vi "Create.vi"(8 "error in (no error)":errorcluster, 11 "ICPCON M7024 in":refnum<class "ICPCON M-7024.lvclass">) -> (0 "error out":errorcluster, 3 "ICPCON M7024 out":refnum<class "ICPCON M-7024.lvclass">)   [LabVIEW 2021, in "ICPCON M-7024.lvclass"]
uses:
  ICPCON M-7024.lvclass
  D:/my_projects/projects/Algorithms/Labview/21/Master CR/Master CR.lvclass
  Data Model/ICPCON ET7000 Data Model/M-7024/M-7024 Data Model.lvclass
  D:/my_projects/projects/Algorithms/Labview/21/Modbus_v121c/Data Model/Device Data Model.lvclass
  Master CR.lvclass/Master CR.ctl
  Serial/Modbus Serial/Modbus Serial.lvclass
  ICPCON M-7024.lvclass/ICPCON M-7024.ctl
  Master CR.lvclass
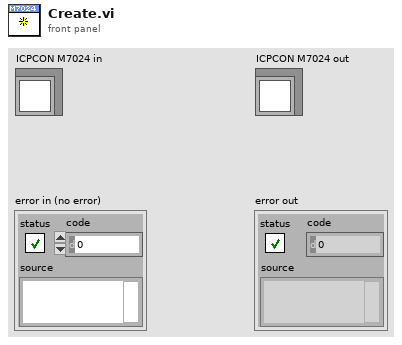
[diagram p1: front panel]
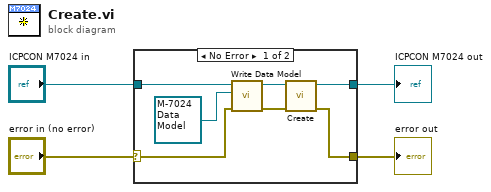
[diagram p0: block diagram]
diagram:
  n1 = case shown="No Error" "error in (no error)" {
    selector: "error in (no error)" -> [w5 w12]
    tunnel: [w9 w12] -> w1
    tunnel: [w10 w13] -> w2
    tunnel: "ICPCON M7024 in" -> [w11 w13]
    frame No Error {
      n2 = call "Write Data Model.vi"("error in (no error)"=w5, "Data Model"=refnum<class "M-7024 Data Model.lvclass"> refnum ("Modbus API:Device Data Model"), "Master CR in"=w11) -> ("error out"=w7:errorcluster, "Master CR out"=w8:refnum<class "ICPCON M-7024.lvclass">)  [unwired: 7 in]
      n3 = call-parent "Create.vi"("error in (no error)"=w7, "Serial in"=w8) -> ("error out"=w9:errorcluster, "Serial out"=w10:refnum<class "ICPCON M-7024.lvclass">)  [unwired: 8 in]
    }
    frame Error {
    }
  }
  "error out" <- w1
  "ICPCON M7024 out" <- w2
